vi "TEST_DSP2.vi"() -> ()   [LabVIEW 2019]
uses:
  _ctrl/DSP_config.ctl
  _ctrl/DSP_retrun.ctl
  _ctrl/create-rw-close.ctl
  _ctrl/DSP_action.ctl
  _ctrl/rw.ctl
panel:
  out "return 2":T1
  out "n":i32
  out "error IO":errorcluster
  in  "config":T2={"Port"="TCPIP0::192.168.0.14::HISLIP0::INSTR", "OVP Level"=0.0, "OCP Level"=0.0, "Current"=0.0, "Voltage"=0.0} {"OCP Level" format="%#_13g"; "OVP Level" format="%#_13g"}
  in  "Exit":bool
  out "VA Chart":cluster{"Data[0]":dbl, "Data[1]":dbl}(graph)
  out "Read Data":string
  in  "connect":bool
  in  "disconntect":bool
  in  "READ":bool
  in  "STOP":bool
  in  "ON":bool
  in  "OFF":bool
  out "error out 3":errorcluster
  # "iDRC"
  # "iDRC DSP1500-30WE"
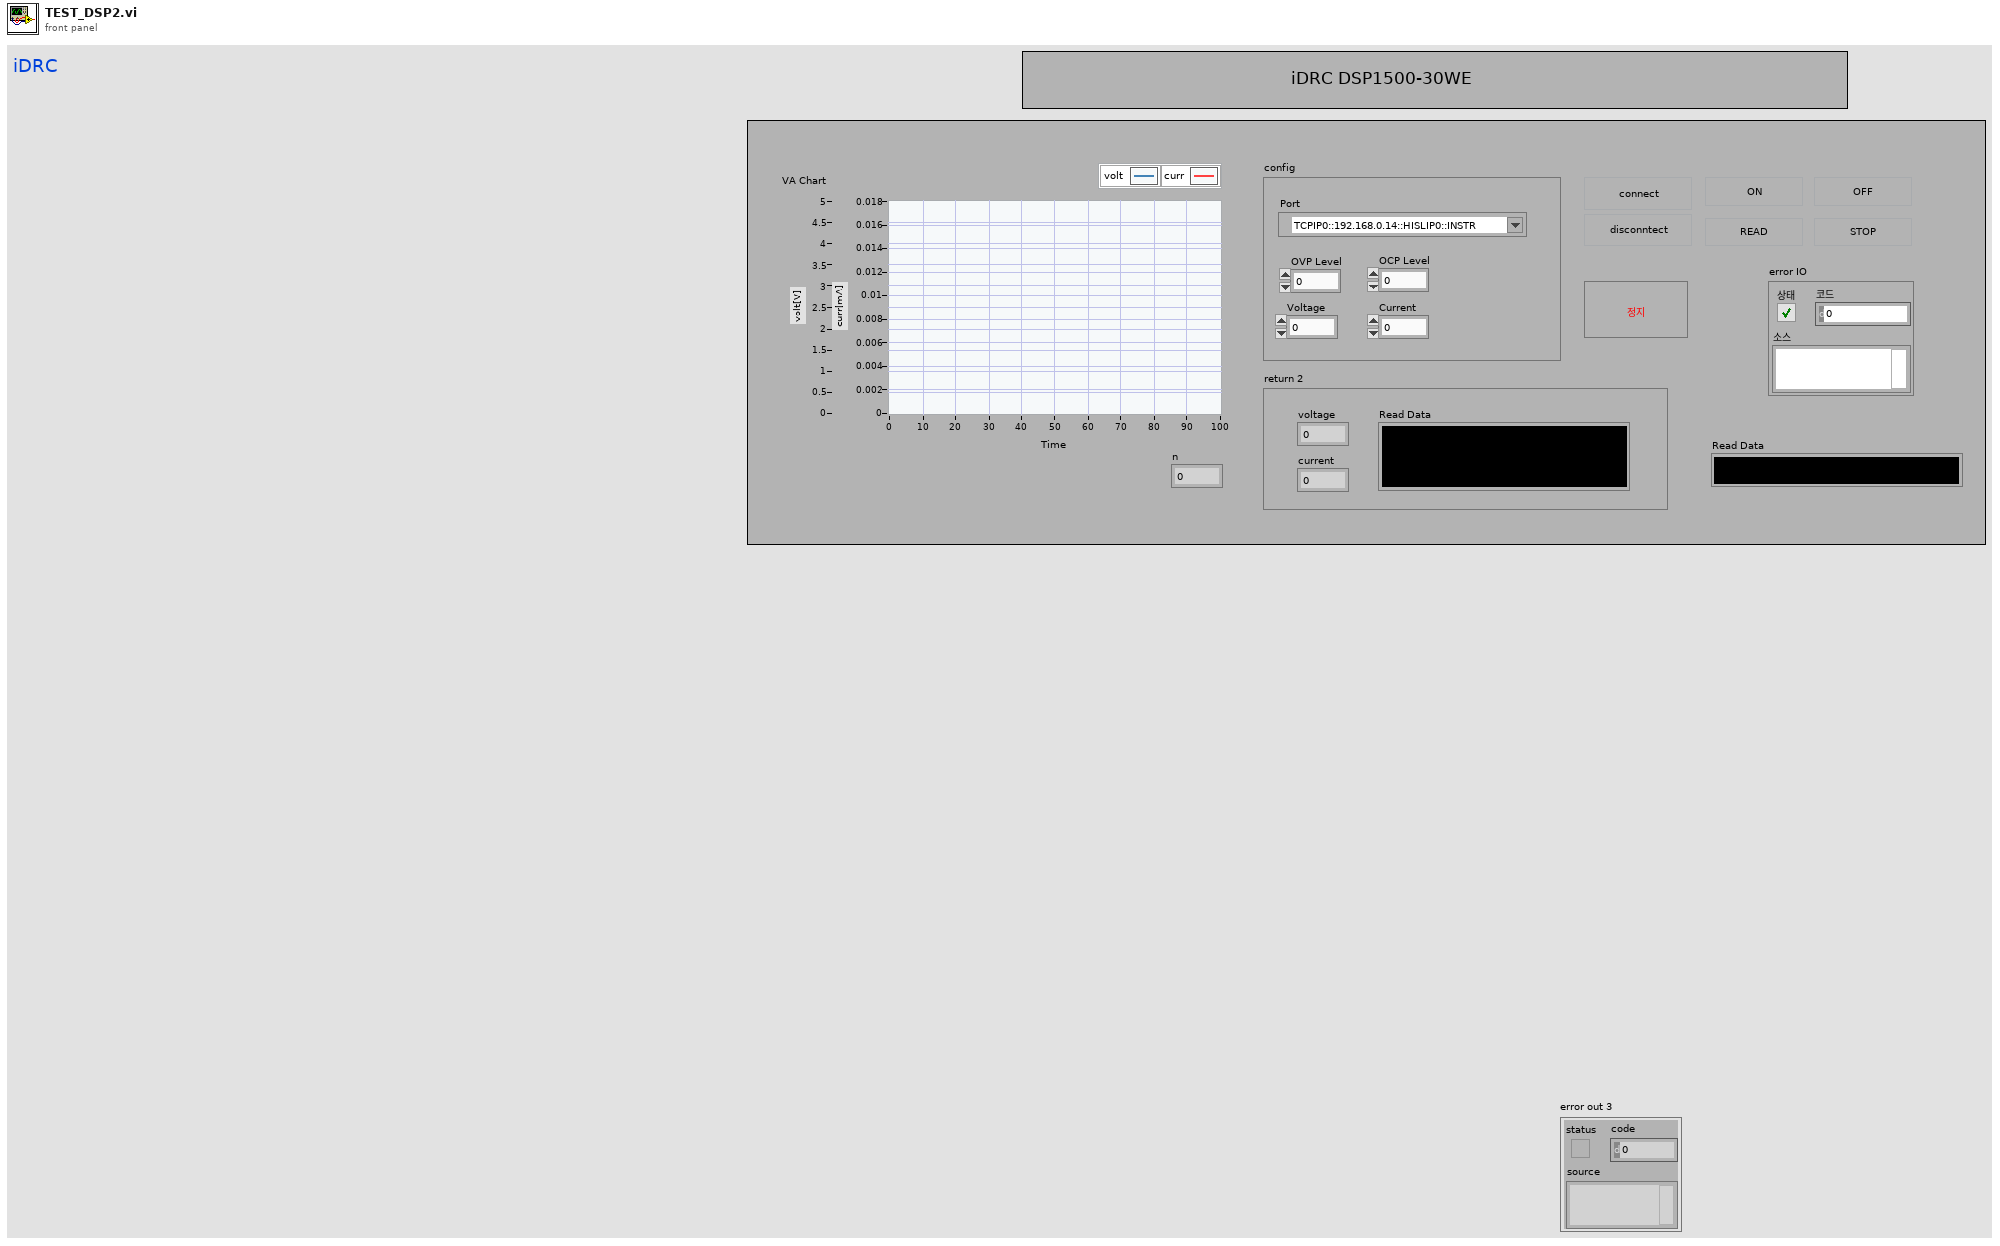
[diagram p1: front panel]
types:
  T1 = typedef "DSP_retrun.ctl" = cluster{"voltage":dbl, "current":dbl, "Read Data":string}
  T2 = typedef "DSP_config.ctl" = cluster{"Port":refnum<visa-resource-name>, "OVP Level":dbl, "OCP Level":dbl, "Current":dbl, "Voltage":dbl}
  T3 = typedef "create-rw-close.ctl" = enum16{"create", "write", "read", "close"}
  T4 = enum8{"Enabled", "Disabled", "Disabled and Grayed Out"}
  T5 = typedef "DSP_action.ctl" = enum16{"False", "cont", "on", "off", "discont", "protection", "preread", "level", "read", "stop", "exit"}
  T6 = typedef "rw.ctl" = enum16{"read", "write"}
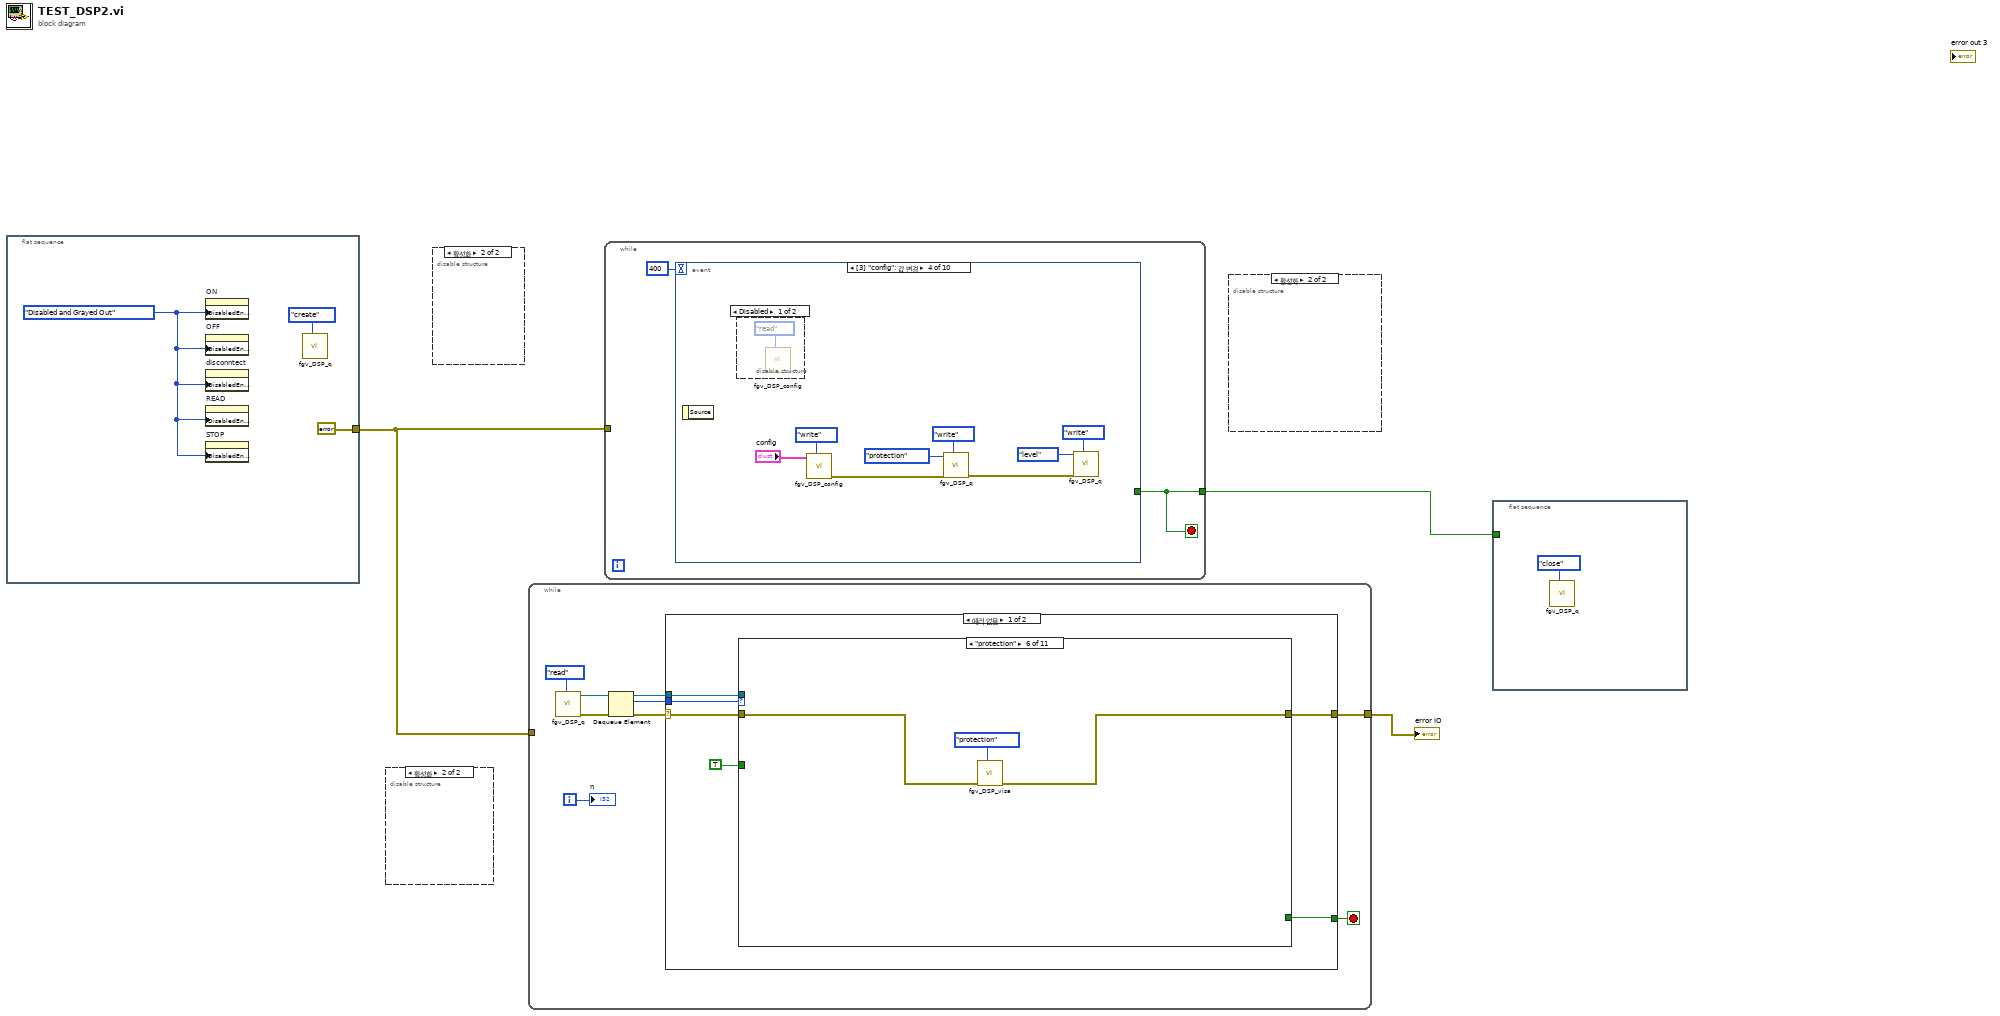
[diagram p0: block diagram]
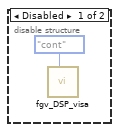
[diagram p2: hidden frame]
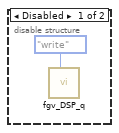
[diagram p3: hidden frame]
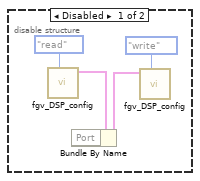
[diagram p4: hidden frame]
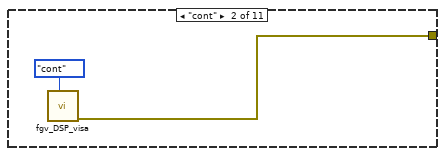
[diagram p6: hidden frame]
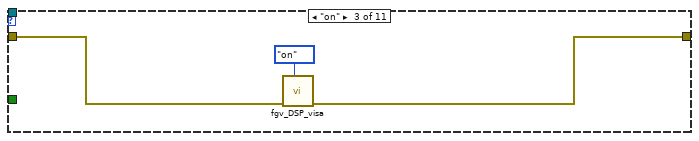
[diagram p7: hidden frame]
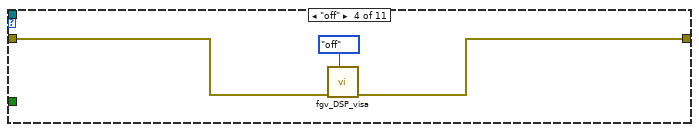
[diagram p8: hidden frame]
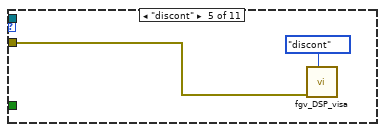
[diagram p9: hidden frame]
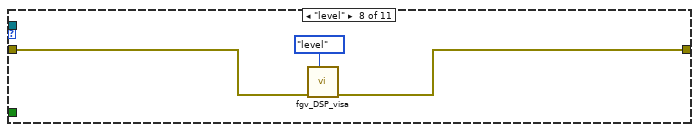
[diagram p11: hidden frame]
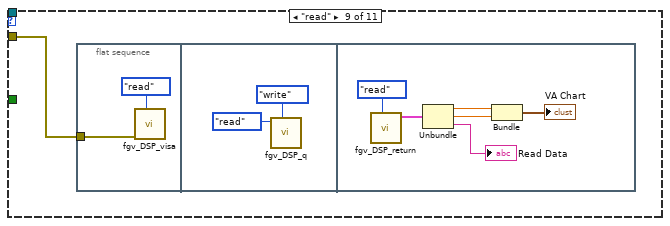
[diagram p12: hidden frame]
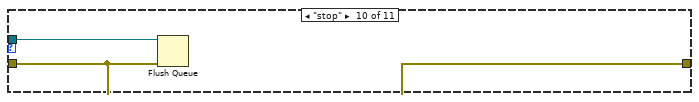
[diagram p13: hidden frame]
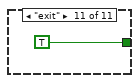
[diagram p14: hidden frame]
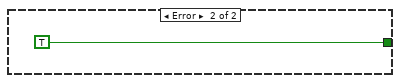
[diagram p15: hidden frame]
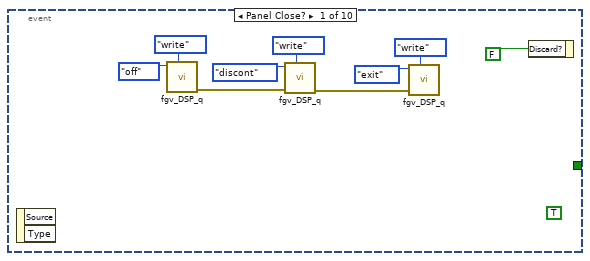
[diagram p16: hidden frame]
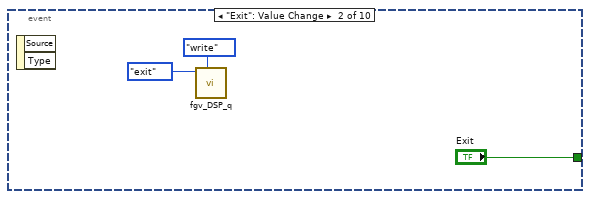
[diagram p17: hidden frame]
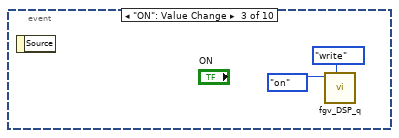
[diagram p18: hidden frame]
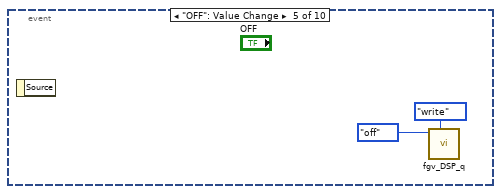
[diagram p20: hidden frame]
diagram:
  n1 = flat-sequence {
    tunnel: [errorcluster {"status"=FALSE, "code"=0, "source"=""} ("에러 출력")] -> w2
    frame #0 {
      w4 = T4."Disabled and Grayed Out" ("비활성화")
      n2 = property on="ON" class="Bool"("DisabledEnum"=w4) -> ()  [unwired: 2 in, 2 out]
      n3 = property on="OFF" class="Bool"("DisabledEnum"=w4) -> ()  [unwired: 2 in, 2 out]
      n4 = property on="disconntect" class="Bool"("DisabledEnum"=w4) -> ()  [unwired: 2 in, 2 out]
      n5 = property on="READ" class="Bool"("DisabledEnum"=w4) -> ()  [unwired: 2 in, 2 out]
      n6 = property on="STOP" class="Bool"("DisabledEnum"=w4) -> ()  [unwired: 2 in, 2 out]
      n7 = call "fgv_DSP_q.vi"("cmd"=create-rw-close."create") -> ()  [unwired: 9 in, 2 out]
    }
  }
  n8 = disable-structure shown="활성화" {
    frame Disabled {
      n9 = call "fgv_DSP_visa.vi"("action"=DSP_action."cont") -> ()  [unwired: 10 in, 1 out]
    }
    frame Enabled {
    }
  }
  n10 = disable-structure shown="활성화" {
    frame Disabled {
      n11 = call "fgv_DSP_q.vi"("cmd"=create-rw-close."write") -> ()  [unwired: 9 in, 2 out]
    }
    frame Enabled {
    }
  }
  n12 = while {
    tunnel: [w16] -> w3
    tunnel: w2 -> [_]
    i -> [w9]
    stop <- w17 stop-if-true
    n13 = call "fgv_DSP_q.vi"("cmd"=create-rw-close."read") -> ("error out"=w14:errorcluster, "queue out"=w13:refnum<queue>)  [unwired: 9 in]
    n14 = Dequeue Element(queue=w13, error in (no error)=w14) -> (queue out=w11:refnum<queue>, element=w12:T5, error out=w10:errorcluster)  [unwired: 1 in, 1 out]
    n15 = case shown="에러 없음" w10 {
      selector: w10 -> [w21 _]
      tunnel: w12 -> [w23 _]
      tunnel: [w20 TRUE] -> w17
      tunnel: w11 -> [w22 _]
      tunnel: [w19 _] -> w16
      frame No Error {
        n16 = case shown="\"protection\"" w23 {
          tunnel: w22 -> [_ _ _ _ _ _ _ _ _ w52 _]
          tunnel: w21 -> [_ _ w27 w30 w32 w36 _ w38 w40 w51 _]
          tunnel: [_ _ _ _ _ _ _ _ _ _ TRUE] -> w20
          tunnel: [_ w24 w26 w29 _ w35 _ w37 _ w51 _] -> w19
          tunnel: TRUE -> [_ _ _ _ _ _ _ _ _ _ _]
          frame "False", Default {
          }
          frame "cont" {
            n17 = call "fgv_DSP_visa.vi"("action"=DSP_action."cont") -> ("error out"=w24:errorcluster)  [unwired: 10 in]
          }
          frame "on" {
            n18 = call "fgv_DSP_visa.vi"("action"=DSP_action."on", "error in"=w27) -> ("error out"=w26:errorcluster)  [unwired: 9 in]
          }
          frame "off" {
            n19 = call "fgv_DSP_visa.vi"("action"=DSP_action."off", "error in"=w30) -> ("error out"=w29:errorcluster)  [unwired: 9 in]
          }
          frame "discont" {
            n20 = call "fgv_DSP_visa.vi"("action"=DSP_action."discont", "error in"=w32) -> ()  [unwired: 9 in, 1 out]
          }
          frame "protection" {
            n21 = call "fgv_DSP_visa.vi"("action"=DSP_action."protection", "error in"=w36) -> ("error out"=w35:errorcluster)  [unwired: 9 in]
          }
          frame "preread" {
          }
          frame "level" {
            n22 = call "fgv_DSP_visa.vi"("action"=DSP_action."level", "error in"=w38) -> ("error out"=w37:errorcluster)  [unwired: 9 in]
          }
          frame "read" {
            n23 = flat-sequence {
              tunnel: w40 -> [w41]
              frame #0 {
                n24 = call "fgv_DSP_visa.vi"("action"=DSP_action."read", "error in"=w41) -> ()  [unwired: 9 in, 1 out]
              }
              frame #1 {
                n25 = call "fgv_DSP_q.vi"("cmd"=create-rw-close."write", "action"=DSP_action."read") -> ()  [unwired: 8 in, 2 out]
              }
              frame #2 {
                n26 = call "fgv_DSP_return.vi"("cmd"=rw."read") -> ("return 2"=w49:T1)  [unwired: 10 in]
                n27 = Unbundle(w49) -> ("voltage"=w46:dbl, "current"=w47:dbl, "Read Data"=→"Read Data":string)
                n28 = Bundle("voltage"=w46, "current"=w47) -> (→"VA Chart":cluster{"voltage":dbl, "current":dbl})  [unwired: 1 in]
              }
            }
          }
          frame "stop" {
            n29 = Flush Queue(queue=w52, error in (no error)=w51) -> ()  [unwired: 3 out]
          }
          frame "exit" {
          }
        }
      }
      frame Error {
      }
    }
    "n" <- w9
  }
  "error IO" <- w3
  n30 = while {
    tunnel: w2 -> [_]
    tunnel: [w55] -> w1
    stop <- w55 stop-if-true
    n31 = event shown="[3] \"config\": 값 변경" {
      selector: _ -> [_ _ _ _ _ _ _ _ _ _]
      dyn-events: _ -> [_ _ _ _ _ _ _ _ _ _]
      timeout: 400 -> [_ _ _ _ _ _ _ _ _ _]
      tunnel: [_ "Exit" _ _ _ _ _ _ _ _] -> w55
      event Panel Close? {
        (unwired) TRUE ("stop")
        n32 = event-data() -> ()  [unwired: 1 in, 2 out]
        n33 = call "fgv_DSP_q.vi"("cmd"=create-rw-close."write", "action"=DSP_action."off") -> ("error out"=w58:errorcluster)  [unwired: 8 in, 1 out]
        n34 = call "fgv_DSP_q.vi"("cmd"=create-rw-close."write", "error in"=w58, "action"=DSP_action."discont") -> ("error out"=w57:errorcluster)  [unwired: 7 in, 1 out]
        n35 = call "fgv_DSP_q.vi"("cmd"=create-rw-close."write", "error in"=w57, "action"=DSP_action."exit") -> ()  [unwired: 7 in, 2 out]
        n36 = event-data("Discard?"=FALSE) -> ()  [unwired: 1 in, 1 out]
      }
      event "Exit": Value Change {
        n37 = event-data() -> ()  [unwired: 1 in, 2 out]
        n38 = call "fgv_DSP_q.vi"("cmd"=create-rw-close."write", "action"=DSP_action."exit") -> ()  [unwired: 8 in, 2 out]
      }
      event "ON": Value Change {
        n39 = event-data() -> ()  [unwired: 1 in, 1 out]
        n40 = call "fgv_DSP_q.vi"("cmd"=create-rw-close."write", "action"=DSP_action."on") -> ()  [unwired: 8 in, 2 out]
      }
      event Value Change {
        n41 = event-data() -> ()  [unwired: 1 in, 1 out]
        n42 = disable-structure shown="Disabled" {
          frame Disabled {
            n43 = call "fgv_DSP_config.vi"("cmd"=rw."read") -> ()  [unwired: 9 in, 2 out]
          }
          frame Enabled {
          }
        }
        n44 = call "fgv_DSP_config.vi"("cmd"=rw."write", "DSP1950 Config"="config") -> ("error out"=w75:errorcluster)  [unwired: 8 in, 1 out]
        n45 = call "fgv_DSP_q.vi"("cmd"=create-rw-close."write", "error in"=w75, "action"=DSP_action."protection") -> ("error out"=w72:errorcluster)  [unwired: 7 in, 1 out]
        n46 = call "fgv_DSP_q.vi"("cmd"=create-rw-close."write", "error in"=w72, "action"=DSP_action."level") -> ()  [unwired: 7 in, 2 out]
      }
      event "OFF": Value Change {
        n47 = event-data() -> ()  [unwired: 1 in, 1 out]
        n48 = call "fgv_DSP_q.vi"("cmd"=create-rw-close."write", "action"=DSP_action."off") -> ()  [unwired: 8 in, 2 out]
      }
      event Timeout {
        n49 = event-data() -> ()  [unwired: 1 in, 1 out]
        n50 = call "fgv_DSP_return.vi"("cmd"=rw."read") -> ("return 2"=→"return 2":T1)  [unwired: 10 in]
      }
      event "READ": Value Change {
        n51 = event-data() -> ()  [unwired: 1 in, 1 out]
        n52 = call "fgv_DSP_q.vi"("cmd"=create-rw-close."write", "action"=DSP_action."read") -> ()  [unwired: 8 in, 2 out]
      }
      event "STOP": Value Change {
        n53 = event-data() -> ()  [unwired: 1 in, 1 out]
        n54 = call "fgv_DSP_q.vi"("cmd"=create-rw-close."write", "action"=DSP_action."stop") -> ()  [unwired: 8 in, 2 out]
      }
      event "connect": Value Change {
        w88 = T4."Enabled" ("비활성화")
        n55 = event-data() -> ("CtlRef"=w92:refnum<vi>)  [unwired: 1 in, 1 out]
        n56 = property class="Bool"(reference=w92) -> ("Label.Text"=w91:string)  [unwired: 1 in, 2 out]
        n57 = call "fgv_DSP_q.vi"("cmd"=create-rw-close."write", "action"=DSP_action."cont") -> ()  [unwired: 8 in, 2 out]
        n58 = case shown="\"conntect\"" w91 {
          frame "False", Default {
          }
          frame "conntect" {
          }
          frame "disconntect" {
          }
        }
        n59 = property on="ON" class="Bool"("DisabledEnum"=w88) -> ()  [unwired: 2 in, 2 out]
        n60 = property on="OFF" class="Bool"("DisabledEnum"=w88) -> ()  [unwired: 2 in, 2 out]
        n61 = property on="disconntect" class="Bool"("DisabledEnum"=w88) -> ()  [unwired: 2 in, 2 out]
        n62 = property on="READ" class="Bool"("DisabledEnum"=w88) -> ()  [unwired: 2 in, 2 out]
        n63 = property on="STOP" class="Bool"("DisabledEnum"=w88) -> ()  [unwired: 2 in, 2 out]
      }
      event "disconntect": Value Change {
        n64 = event-data() -> ()  [unwired: 1 in, 1 out]
        n65 = call "fgv_DSP_q.vi"("cmd"=create-rw-close."write", "action"=DSP_action."discont") -> ()  [unwired: 8 in, 2 out]
      }
    }
  }
  n66 = disable-structure shown="활성화" {
    frame Disabled {
      n67 = call "fgv_DSP_config.vi"("cmd"=rw."read") -> ("DSP1950 Config 2"=w97:T2)  [unwired: 9 in, 1 out]
      n68 = Bundle By Name(cluster=w97) -> (w98:T2)  [unwired: 1 in]
      n69 = call "fgv_DSP_config.vi"("cmd"=rw."write", "DSP1950 Config"=w98) -> ()  [unwired: 8 in, 2 out]
    }
    frame Enabled {
    }
  }
  n70 = flat-sequence {
    tunnel: w1 -> [_]
    frame #0 {
      n71 = call "fgv_DSP_q.vi"("cmd"=create-rw-close."close") -> ()  [unwired: 9 in, 2 out]
    }
  }
